vi "FinalCalc.vi"(11 "Prop":T1[](array[typedef])) -> (3 "Prop out":T1={"Raw Data"=[[0.0], [0.0234375], [0.9609375]], "Poperties"={"RMS values"=[], "Max"=[], "Min"=[], "A(8)"=[], "t"=0.0, "A(8) Axis"=0.0, "Aw"=[], "Ak 30min"=0.0, "Ak_axis"=0, "Spec"=[]}, "Power Spectrum / PSD"=[]})   [LabVIEW 2019]
uses:
  Communication/TypeDef/#TypeDef_PropGraph.ctl
  Communication/TypeDef/#TypeDef_PropertiesToSave.ctl
panel:
  in  "PropGraph":T1={"Raw Data"=[[0.0], [0.0234375], [0.9609375]], "Poperties"={"RMS values"=[], "Max"=[], "Min"=[], "A(8)"=[], "t"=0.0, "A(8) Axis"=0.0, "Aw"=[], "Ak 30min"=0.0, "Ak_axis"=0, "Spec"=[]}, "Power Spectrum / PSD"=[]}
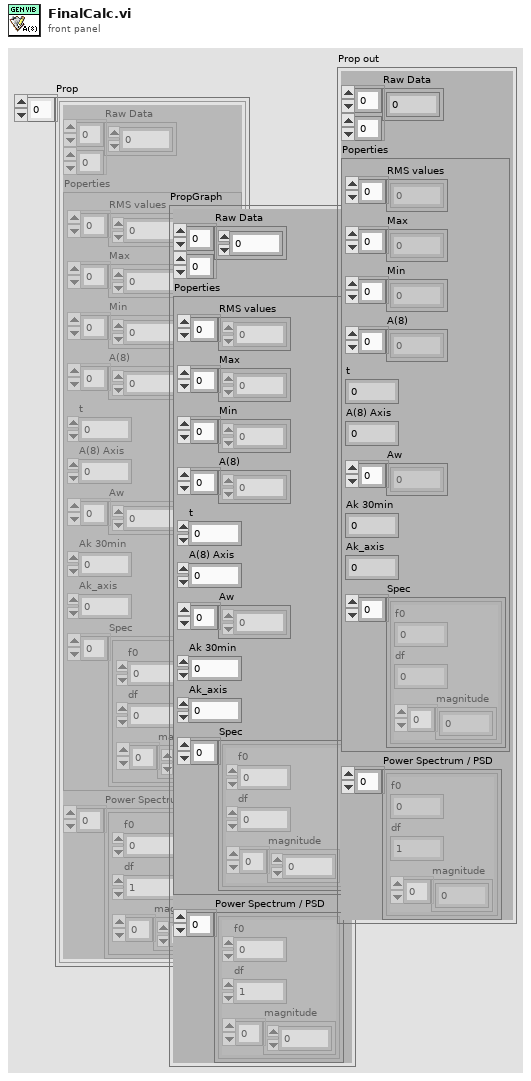
[diagram p1: front panel]
types:
  T1 = typedef "#TypeDef_PropGraph.ctl" = cluster{"Raw Data":dbl[][], "Poperties":T2, "Power Spectrum / PSD":cluster{"f0":dbl, "df":dbl, "magnitude":dbl[]}[]}
  T2 = typedef "#TypeDef_PropertiesToSave.ctl" = cluster{"RMS values":dbl[], "Max":dbl[], "Min":dbl[], "A(8)":dbl[], "t":dbl, "A(8) Axis":dbl, "Aw":dbl[], "Ak 30min":dbl, "Ak_axis":i32, "Spec":cluster{"f0":dbl, "df":dbl, "magnitude":dbl[]}[]}
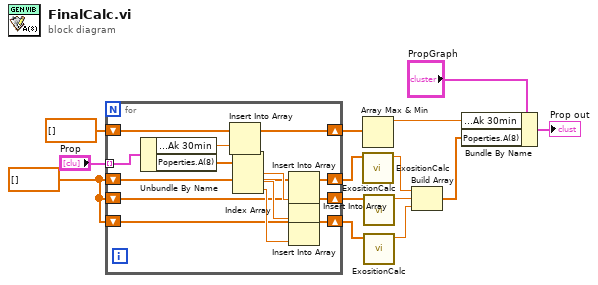
[diagram p0: block diagram]
diagram:
  w8 = dbl[] []
  n1 = for {
    tunnel: "Prop" -> [w28] mode=indexing
    shift-right: [w22] -> w7
    shift-left: w8 -> [w17]
    shift-right: [w26] -> w13
    shift-left: dbl[] [] -> [w25]
    shift-right: [w19] -> w6
    shift-left: w8 -> [w16]
    shift-right: [w18] -> w5
    shift-left: w8 -> [w15]
    n2 = Unbundle By Name(w28) -> ("Poperties.Ak 30min"=w27:dbl, "Poperties.A(8)"=w24:dbl[])
    n3 = Insert Into Array(array=w25, new element=w27) -> (w26:dbl[])  [unwired: 1 in]
    n4 = Index Array(array=w24) -> (element #1=w23:dbl, element #2=w21:dbl, element #3=w20:dbl)  [unwired: 3 in]
    n5 = Insert Into Array(array=w17, new element=w23) -> (w22:dbl[])  [unwired: 1 in]
    n6 = Insert Into Array(array=w16, new element=w21) -> (w19:dbl[])  [unwired: 1 in]
    n7 = Insert Into Array(array=w15, new element=w20) -> (w18:dbl[])  [unwired: 1 in]
  }
  n8 = Array Max & Min(array=w13) -> (max value=w10:dbl)  [unwired: 3 out]
  n9 = call "ExositionCalc.vi"("A(8)axis"=w7) -> ("A(8)axis"=w4:dbl)  [unwired: 10 in]
  n10 = call "ExositionCalc.vi"("A(8)axis"=w6) -> ("A(8)axis"=w3:dbl)  [unwired: 10 in]
  n11 = call "ExositionCalc.vi"("A(8)axis"=w5) -> ("A(8)axis"=w2:dbl)  [unwired: 10 in]
  n12 = Build Array(w4, w3, w2) -> (w1:dbl[])
  n13 = Bundle By Name(cluster="PropGraph", "Poperties.Ak 30min"=w10, "Poperties.A(8)"=w1) -> (→"Prop out":T1)
